vi "DMM Cfg Multi Point - Continuous.vi"(8 "error in (no error)":errorcluster, 10 "JSONCluster":T1 {"DMMVoltageFaultUpperLimit" format="%#_6p"}, 11 "IVI Refnum in":refnum<k15>) -> (0 "error out":errorcluster, 3 "IVI Refnum out":refnum<k15>)   [LabVIEW 2019]
uses:
  JSONCluster.ctl
  <instrlib>/niDMM/nidmm.llb/niDMM Sample Trigger.ctl
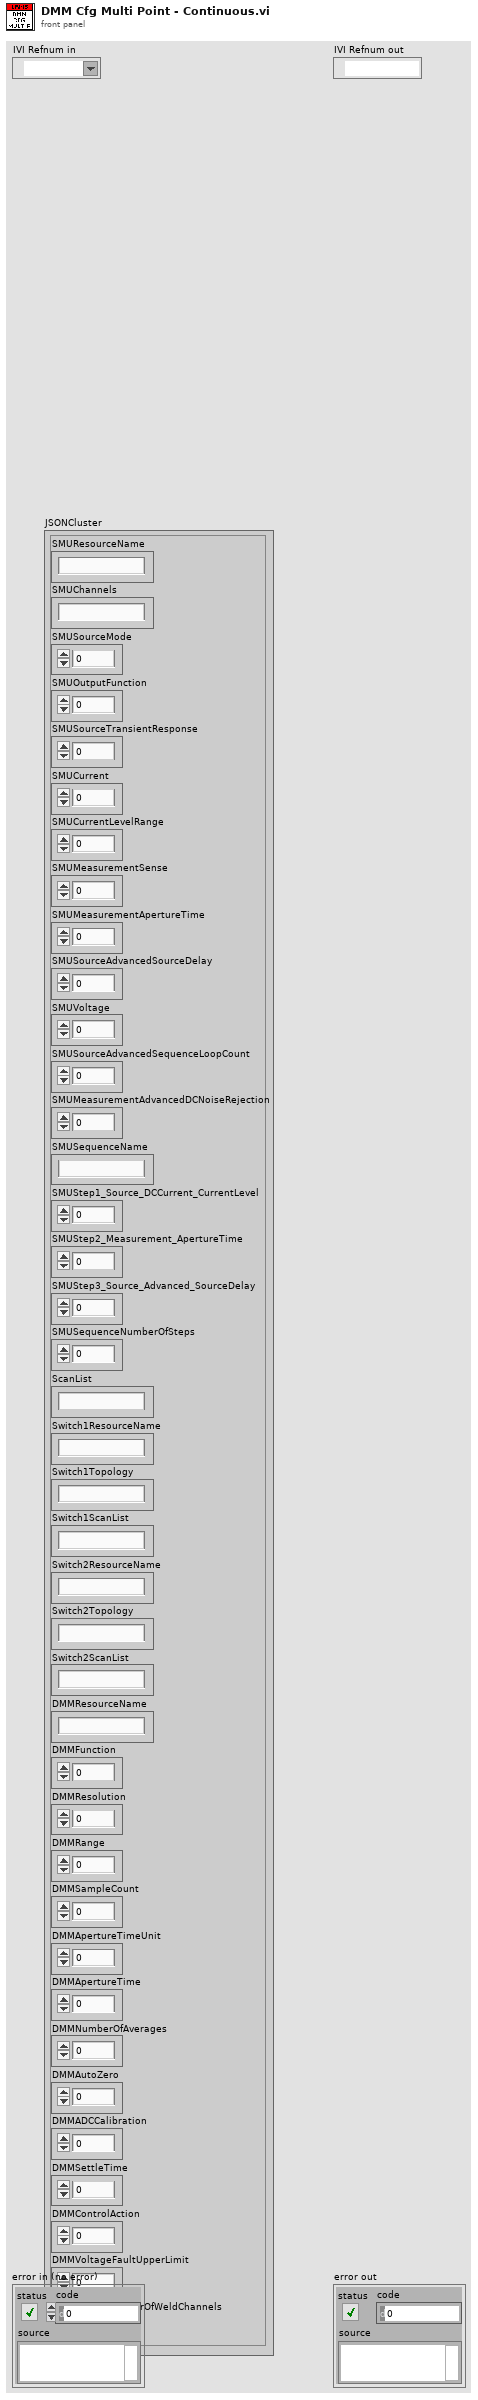
[diagram p1: front panel]
types:
  T1 = typedef "JSONCluster.ctl" = cluster{"SMUResourceName":string, "SMUChannels":string, "SMUSourceMode":i32, "SMUOutputFunction":i32, "SMUSourceTransientResponse":i32, "SMUCurrent":dbl, "SMUCurrentLevelRange":dbl, "SMUMeasurementSense":i32, "SMUMeasurementApertureTime":dbl, "SMUSourceAdvancedSourceDelay":dbl, "SMUVoltage":dbl, "SMUSourceAdvancedSequenceLoopCount":i32, "SMUMeasurementAdvancedDCNoiseRejection":i32, "SMUSequenceName":string, "SMUStep1_Source_DCCurrent_CurrentLevel":i32, "SMUStep2_Measurement_ApertureTime":i32, "SMUStep3_Source_Advanced_SourceDelay":i32, "SMUSequenceNumberOfSteps":i32, "ScanList":string, "Switch1ResourceName":string, "Switch1Topology":string, "Switch1ScanList":string, "Switch2ResourceName":string, "Switch2Topology":string, "Switch2ScanList":string, "DMMResourceName":string, "DMMFunction":i32, "DMMResolution":dbl, "DMMRange":dbl, "DMMSampleCount":i32, "DMMApertureTimeUnit":i32, "DMMApertureTime":dbl, "DMMNumberOfAverages":i32, "DMMAutoZero":i32, "DMMADCCalibration":i32, "DMMSettleTime":dbl, "DMMControlAction":i32, "DMMVoltageFaultUpperLimit":dbl, "ApplicationNumberOfWeldChannels":i32}
  T2 = typedef "niDMM Sample Trigger.ctl" = enum16{"Immediate", "External", "TTL 0", "TTL 1", "TTL 2", "TTL 3", "TTL 4", "TTL 5", "TTL 6", "Interval", "Software", "TTL 7", "PXI Star", "LBR Trig 1", "Aux Trig 1"}
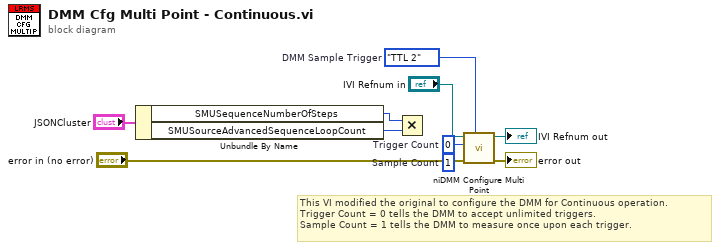
[diagram p0: block diagram]
diagram:
  w1 = 1  # Sample Count
  w2 = 0  # Trigger Count
  w3 = niDMM_Sample_Trigger."TTL 2"  # DMM Sample Trigger
  # "This VI modified the original to configure the DMM for Continuous operation.\nTrigger Count = 0 tells the DMM to accept unlimited triggers.\nSample Count = 1 tells the DMM to measure once upon each trigger."
  n1 = Unbundle By Name("JSONCluster") -> ("SMUSequenceNumberOfSteps"=w8:i32, "SMUSourceAdvancedSequenceLoopCount"=w9:i32)
  n2 = Multiply(x=w8, y=w9) -> ()  [unwired: 1 out]
  n3 = call <instrlib>:"niDMM Configure Multi Point.vi"("Sample Trigger"=w3, "error in (no error)"="error in (no error)", "Sample Count"=w1, "Trigger Count"=w2, "instrument handle"="IVI Refnum in") -> ("error out"=→"error out":errorcluster, "instrument handle out"=→"IVI Refnum out":refnum<k15>)  [unwired: 5 in]
